vi "Set Menu Properties.vi"(6 "menu reference":refnum<k9>, 8 "Menu Tag":string[](array[string]), 9 "enabled":bool, 11 "error in (no error)":errorcluster) -> (3 "error out":errorcluster)   [LabVIEW 2014]
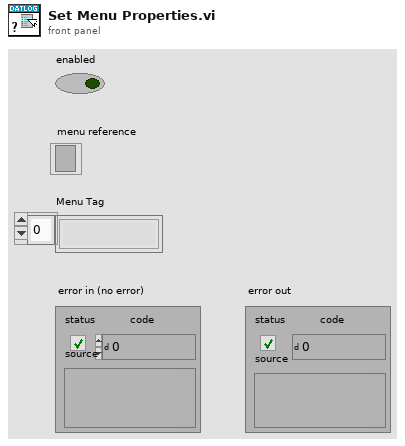
[diagram p1: front panel]
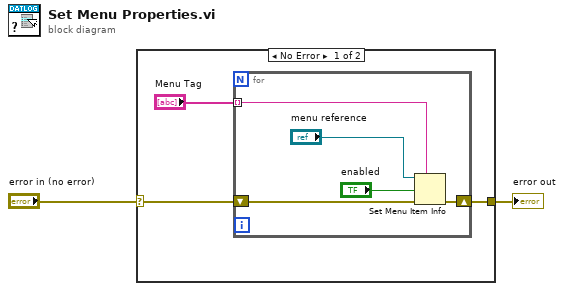
[diagram p0: block diagram]
diagram:
  n1 = case shown="No Error" "error in (no error)" {
    selector: "error in (no error)" -> [w4 w11]
    tunnel: [w3 w11] -> w1
    frame No Error {
      n2 = for {
        tunnel: "Menu Tag" -> [w6] mode=indexing
        shift-right: [w8] -> w3
        shift-left: w4 -> [w9]
        n3 = Set Menu Item Info(7:w6, 8:w9, 9:"enabled", 11:"menu reference") -> (0:w8:errorcluster)  [unwired: 3 in, 1 out]
      }
    }
    frame Error {
    }
  }
  "error out" <- w1
